vi "Teleop.vi"(10 "Match Info":T1={"Autonomous Elapsed Seconds"=0.0, "TeleOp Elapsed Seconds"=0.0, "Disabled Elapsed Seconds"=0.0, "Visited Autonomous"=FALSE, "Visited TeleOp"=FALSE, "Visited Disabled"=FALSE, "Autonomous Settings"={"Autonomous Style"=enum."Independent", "VI Refnum"=refnum}}, 11 "Call Context":T2) -> ()   [LabVIEW 2018]
doc: "This VI is called for each TeleOp packet received from the DS where the robot is not disabled. It is often used to read from the joysticks and update I/O or to update setpoints for timed control loops. It should complete and return within 20 milliseconds or it may miss DS packets."
uses:
  <vilib>/Rock Robotics/WPI/DriverStation/WPI_DriverStationDerivedRobotMode.ctl
  <vilib>/Rock Robotics/WPI/DriverStation/WPI_DriverStationMatch Info.ctl
  DeepSpaceSrc/Global_Var-RefNum/Joystick_Control.vi
  ArgosLib/ArgosLib.lvlib
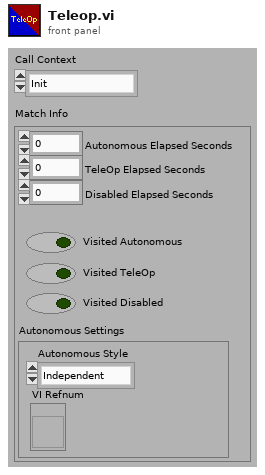
[diagram p1: front panel]
types:
  T1 = typedef "WPI_DriverStationMatch Info.ctl" = cluster{"Autonomous Elapsed Seconds":dbl, "TeleOp Elapsed Seconds":dbl, "Disabled Elapsed Seconds":dbl, "Visited Autonomous":bool, "Visited TeleOp":bool, "Visited Disabled":bool, "Autonomous Settings":cluster{"Autonomous Style":enum16{"Iterative", "Independent"}, "VI Refnum":refnum<vi>}}
  T2 = typedef "WPI_DriverStationDerivedRobotMode.ctl" = enum16{"Init", "Execute", "Stop"}
  T3 = typedef "RobotJoysticks.ctl" = cluster{"Driver Controller":T4, "Operator Controller":T4}
  T4 = typedef "WPI_JoystickDevRef.ctl" = cluster{"Device":T5}
  T5 = typedef "WPI_JoystickDeviceEnum.ctl" = enum16{"USB 0", "USB 1", "USB 2", "USB 3", "USB 4", "USB 5"}
  T6 = typedef "ArgosLib.lvlib/XBoxAxes_Type.ctl" = cluster{"Left_Trigger":dbl, "Right_Trigger ":dbl, "Left_X":dbl, "Left_Y":dbl, "Right_X":dbl, "Right_Y":dbl}
  T7 = typedef "ArgosLib.lvlib/XBoxButtons_Type.ctl" = cluster{"A":bool, "B":bool, "X":bool, " Y":bool, "LB":bool, " RB":bool, "Left_Thumb_Button":bool, "Right_Thumb_Button":bool, "Back":bool, "Start":bool, "Top":bool, "Right":bool, "Bottom":bool, "Left":bool}
  T8 = typedef "JoystickControls.ctl" = cluster{"Unassigned_LY":dbl, "Unassigned_RX":dbl, "Unassigned_LX":dbl, "Unassigned_RY":dbl, "Unassigned_A":bool, "Unassigned_RT":dbl, "Unassigned_LT":dbl, "Unassigned_B":bool, "Unassigned_X":bool, "Unassigned_Y":bool, "Unassigned_LB":bool, "Unassigned_RB":bool, "Unassigned_LJ":bool, "Unassigned_RJ":bool, "Swap_Back":bool, "Swap_Start":bool, "Unassigned_LY 2":dbl, "Unassigned_RX 2":dbl, "Unassigned_LX 2":dbl, "Unassigned_RY 2":dbl, "Unassigned_A 2":bool, "Unassigned_RT 2":dbl, "Unassigned_LT 2":dbl, "Unassigned_B 2":bool, "Unassigned_X 2":bool, "Unassigned_Y 2":bool, "Unassigned_LB 2":bool, "Unassigned_RB 2":bool, "Unassigned_LJ 2":bool, "Unassigned_RJ 2":bool, "Swap_Back 2":bool, "Swap_Start 2":bool, "Unassigned_Up 2":bool, "Unassigned_Right 2":bool, "Unassigned_Down 2":bool, "Unassigned_Left 2":bool, "Unassigned_Up":bool, " Unassigned_Right":bool, "Unassigned_Down":bool, "Unassigned_Left":bool}
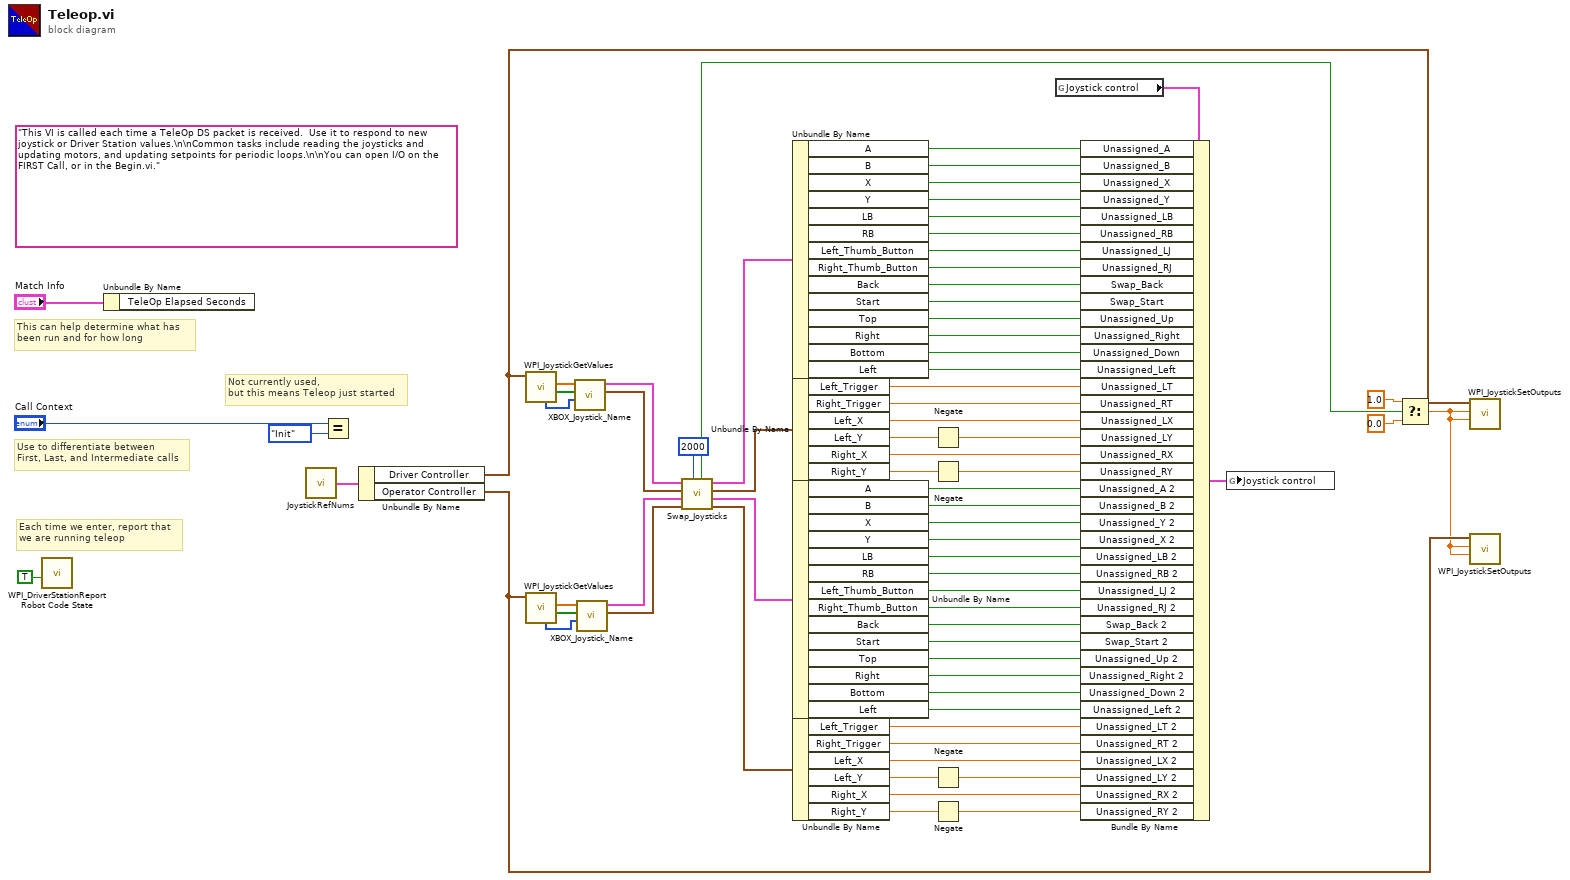
[diagram p0: block diagram]
diagram:
  (unwired) "This VI is called each time a TeleOp DS packet is received.  Use it to respond to new joystick or Driver Station values.\n\nCommon tasks include reading the joysticks and updating motors, and updating setpoints for periodic loops.\n\nYou can open I/O on the FIRST Call, or in the Begin.vi."
  # "Not currently used,\nbut this means Teleop just started"
  # "Each time we enter, report that\nwe are running teleop"
  # "Use to differentiate between\nFirst, Last, and Intermediate calls"
  # "This can help determine what has\nbeen run and for how long"
  n1 = call <vilib>:"WPI_DriverStationReport Robot Code State.vi"("TeleOp"=TRUE ("Autonomous")) -> ()  [unwired: 10 in, 1 out]
  n2 = Unbundle By Name("Match Info") -> ()  [unwired: 1 out]
  n3 = call "JoystickRefNums.vi"() -> ("Joysticks"=w68:T3)  [unwired: 1 in]
  n4 = Equal?(x="Call Context", y=WPI_DriverStationDerivedRobotMode."Init") -> ()  [unwired: 1 out]
  n5 = Unbundle By Name(w68) -> ("Driver Controller"=w6:T4, "Operator Controller"=w5:T4)
  n6 = call <vilib>:"WPI_JoystickGetValues.vi"("JoystickDevRef"=w6) -> ("Buttons"=w66:bool[], "Axes"=w67:dbl[], "POVs"=w65:i16[])  [unwired: 6 in, 2 out]
  n7 = call <vilib>:"WPI_JoystickGetValues.vi"("JoystickDevRef"=w5) -> ("Buttons"=w63:bool[], "Axes"=w64:dbl[], "POVs"=w62:i16[])  [unwired: 6 in, 2 out]
  n8 = call "XBOX_Joystick_Name.vi"("POVs"=w65, "Buttons"=w66, "Axes"=w67) -> ("Named Axes"=w60:T6, "Named Buttons"=w61:T7)  [unwired: 7 in]
  n9 = call "XBOX_Joystick_Name.vi"("POVs"=w62, "Buttons"=w63, "Axes"=w64) -> ("Named Axes"=w58:T6, "Named Buttons"=w59:T7)  [unwired: 7 in]
  n10 = call "Swap_Joysticks.vi"("Hold Time(ms)"=u32 2000, "Axes 1 In"=w58, "Buttons 1"=w59, "Axes 0 in"=w60, "Buttons 0"=w61) -> ("Axes 1 out"=w53:T6, "Buttons 1 out"=w54:T7, "Axes 0 out"=w55:T6, "Buttons 0 Out"=w56:T7, "Swap?"=w3:bool)
  n11 = Unbundle By Name(w56) -> ("A"=w52:bool, "B"=w50:bool, "X"=w49:bool, "Y"=w48:bool, "LB"=w47:bool, "RB"=w46:bool, "Left_Thumb_Button"=w45:bool, "Right_Thumb_Button"=w44:bool, "Back"=w43:bool, "Start"=w42:bool, "Top"=w41:bool, "Right"=w40:bool, "Bottom"=w39:bool, "Left"=w38:bool)
  n12 = Unbundle By Name(w55) -> ("Left_Trigger"=w37:dbl, "Right_Trigger"=w36:dbl, "Left_X"=w35:dbl, "Left_Y"=w34:dbl, "Right_X"=w33:dbl, "Right_Y"=w32:dbl)
  n13 = Unbundle By Name(w54) -> ("A"=w31:bool, "B"=w30:bool, "X"=w29:bool, "Y"=w28:bool, "LB"=w27:bool, "RB"=w26:bool, "Left_Thumb_Button"=w25:bool, "Right_Thumb_Button"=w24:bool, "Back"=w23:bool, "Start"=w22:bool, "Top"=w21:bool, "Right"=w20:bool, "Bottom"=w19:bool, "Left"=w18:bool)
  n14 = Unbundle By Name(w53) -> ("Left_Trigger"=w17:dbl, "Right_Trigger"=w16:dbl, "Left_X"=w15:dbl, "Left_Y"=w14:dbl, "Right_X"=w13:dbl, "Right_Y"=w12:dbl)
  n15 = Negate(x=w34) -> (-x=w11:dbl)
  n16 = Negate(x=w32) -> (-x=w10:dbl)
  n17 = Negate(x=w14) -> (-x=w9:dbl)
  n18 = Negate(x=w12) -> (-x=w8:dbl)
  n19 = global read "Joystick_Control.vi" "Joystick control"() -> (w51:T8)
  n20 = Bundle By Name(cluster=w51, "Unassigned_A"=w52, "Unassigned_B"=w50, "Unassigned_X"=w49, "Unassigned_Y"=w48, "Unassigned_LB"=w47, "Unassigned_RB"=w46, "Unassigned_LJ"=w45, "Unassigned_RJ"=w44, "Swap_Back"=w43, "Swap_Start"=w42, "Unassigned_Up"=w41, "Unassigned_Right"=w40, "Unassigned_Down"=w39, "Unassigned_Left"=w38, "Unassigned_LT"=w37, "Unassigned_RT"=w36, "Unassigned_LX"=w35, "Unassigned_LY"=w11, "Unassigned_RX"=w33, "Unassigned_RY"=w10, "Unassigned_A 2"=w31, "Unassigned_B 2"=w30, "Unassigned_Y 2"=w29, "Unassigned_X 2"=w28, "Unassigned_LB 2"=w27, "Unassigned_RB 2"=w26, "Unassigned_LJ 2"=w25, "Unassigned_RJ 2"=w24, "Swap_Back 2"=w23, "Swap_Start 2"=w22, "Unassigned_Up 2"=w21, "Unassigned_Right 2"=w20, "Unassigned_Down 2"=w19, "Unassigned_Left 2"=w18, "Unassigned_LT 2"=w17, "Unassigned_RT 2"=w16, "Unassigned_LX 2"=w15, "Unassigned_LY 2"=w9, "Unassigned_RX 2"=w13, "Unassigned_RY 2"=w8) -> (w7:T8)
  n21 = global write "Joystick_Control.vi" "Joystick control"(w7) -> ()
  n22 = Select(t=sgl 1.0, s=w3, f=sgl 0.0) -> (s? t:f=w4:sgl)
  n23 = call <vilib>:"WPI_JoystickSetOutputs.vi"("Right Rumble"=w4, "Left Rumble"=w4, "JoystickDevRef"=w6) -> ()  [unwired: 7 in, 2 out]
  n24 = call <vilib>:"WPI_JoystickSetOutputs.vi"("Right Rumble"=w4, "Left Rumble"=w4, "JoystickDevRef"=w5) -> ()  [unwired: 7 in, 2 out]
